vi "Channel Probe.vi"(2 "channelOp":enum16{"init", "write", "read", "probe"}(ring), 3 "PipeData in":refnum<class "StreamData.lvclass">) -> (1 "PipeData out":refnum<class "StreamData.lvclass">)   [LabVIEW 2017, in "Stream-t'WPI_EncoderType.ctl'.lvlib"]
doc: "Displays the status of the channel as the channel is modified by the various endpoints and gives the user ways to pause the application using the channel."
uses:
  <extravilib>/ChannelInstances/Stream-t'WPI_EncoderType.ctl'.lvlib
  <extravilib>/ChannelInstances/Stream-t'WPI_EncoderType.ctl'/StreamData.lvclass
  <vilib>/Rock Robotics/WPI/Encoder/WPI_EncoderType.ctl
  <extravilib>/ChannelInstances/Stream-t'WPI_EncoderType.ctl'/ChannelOp.ctl
  <vilib>/Utility/miscctls.llb/LVPositionTypeDef.ctl
panel:
  in  "Details":string="Details"
  in  "Operation Count":string="Operation Count:"
  out "Details":string
  in  "Last Operation":string="Last Operation:"
  in  "Read":string="Read"
  in  "Write":string="Write"
  in  "Single Step":bool
  in  "Element To Match":T1
  in  "Pause when latest element matches":bool
  in  "Pause when aborted":bool
  in  "Pause when last element written":bool
  in  "Fixed Size":string="<b>Current Element Count:</b>\n%d\n<b>Allocated Element Count:</b>\n%d (Fixed Size)\n"
  in  "Unbounded":string="<b>Current Element Count:</b>\n%d\n<b>Allocated Element Count:</b>\n%d (Unbounded)\n"
  out "Details":string
  in  "Play":bool
  out "Aborted?":bool
  out "Last element written?":bool
  in  "Pause":bool
  out "No Endpoiont Yet":string="\n\n\n\n\n\n\n\n\n\n\nNeither endpoint has executed yet."
  out "Latest":string="Latest\nEnqueue"
  out "Next":string="Next\nDequeue"
  out "Stream Data":cluster{"element":T1}[](array[cluster])
  # "Details"
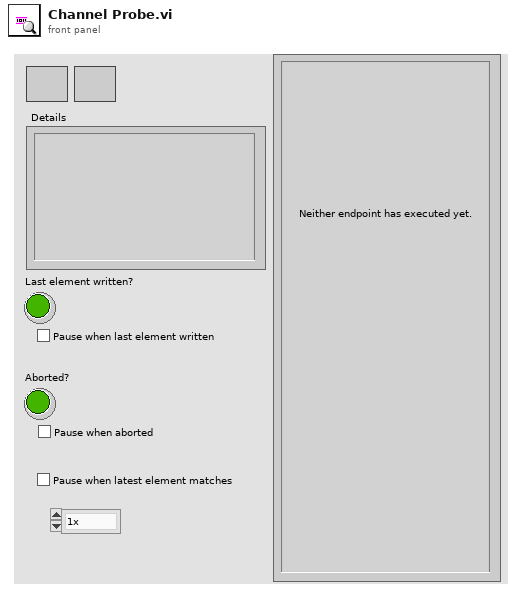
[diagram p1: front panel]
types:
  T1 = typedef "WPI_EncoderType.ctl" = enum16{"1x", "2x", "4x"}
  T2 = typedef "Stream-t'WPI_EncoderType.ctl'.lvlib/ChannelOp.ctl" = enum16{"init", "write", "read", "probe"}
  T3 = enum32{"Invalid", "Standard", "Closed", "Hidden", "Minimized", "Maximized"}
  T4 = typedef "LVPositionTypeDef.ctl" = cluster{"Left":i32, "Top":i32}
  T5 = typedef "LVPointTypeDef.ctl" = cluster{"Horizontal":i16, "Vertical":i16}
  T6 = typedef "LVBoundsTypeDef.ctl" = cluster{"Width":u32, "Height":u32}
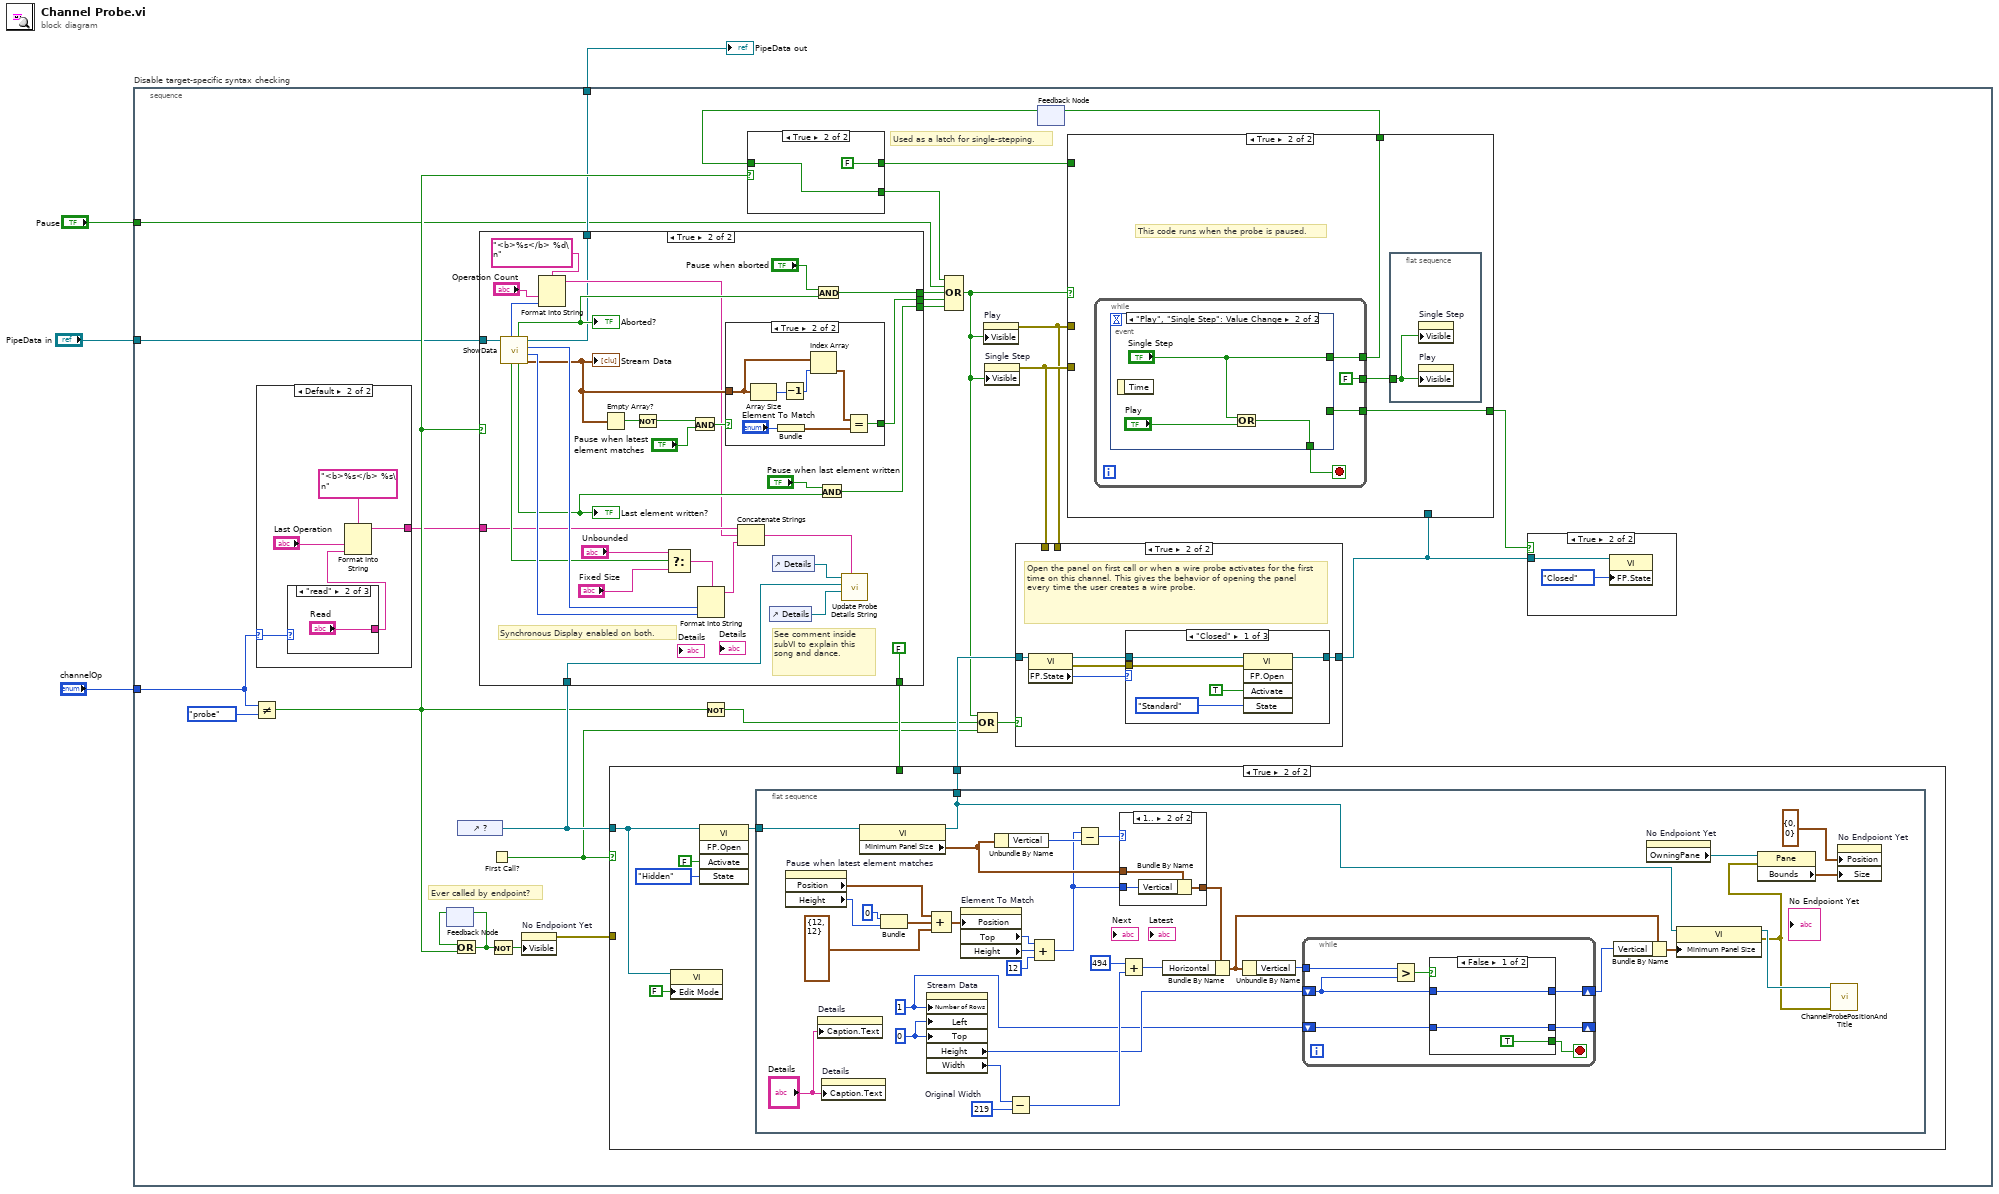
[diagram p0: block diagram]
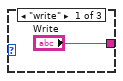
[diagram p3: hidden frame]
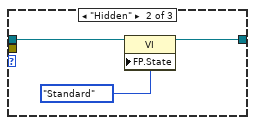
[diagram p7: hidden frame]
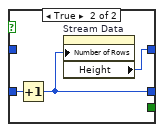
[diagram p12: hidden frame]
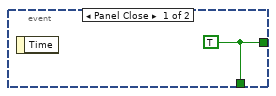
[diagram p15: hidden frame]
diagram:
  n1 = stacked-sequence "Disable target-specific syntax checking" {
    tunnel: "PipeData in" -> [w8]
    tunnel: [w7] -> w3
    tunnel: "Pause" -> [w6]
    tunnel: "channelOp" -> [w5]
    frame #0 {
      # "Used as a latch for single-stepping."
      # "Ever called by endpoint?"
      n2 = Not Equal?(x=w5, y=ChannelOp."probe" ("channelOp 2")) -> (x != y?=w15:bool)
      n3 = case shown="Default" w5 {
        selector: w5 -> [_ w38]
        tunnel: [_ w36] -> w11
        frame "init", "probe" {
        }
        frame Default {
          n4 = case shown="\"read\"" w38 {
            tunnel: ["Write" "Read" _] -> w35
            frame "write" {
            }
            frame "read" {
            }
            frame Default {
            }
          }
          n5 = Format Into String(format string="<b>%s</b> %s\n", "Last Operation", w35) -> (resulting string=w36:string)  [unwired: 2 in, 1 out]
        }
      }
      n6 = feedback #1() -> (w27:bool)  [unwired: 1 in]
      n7 = Or(x=w27, y=w15) -> (x .or. y?=w26:bool)
      n8 = feedback-in #1(w26) -> ()
      n9 = control-ref of="?"() -> (w28:refnum<vi>)
      n10 = case shown="True" w15 {
        tunnel: w8 -> [w59 w84]
        tunnel: [_ w79] -> w32
        tunnel: [_ w73] -> w31
        tunnel: [_ w72] -> w30
        tunnel: [_ FALSE ("always false")] -> w29
        tunnel: w28 -> [_ w70]
        tunnel: w11 -> [_ w69]
        tunnel: [w59 w60] -> w7
        frame False {
        }
        frame True {
          # "See comment inside subVI to explain this song and dance."
          # "Synchronous Display enabled on both."
          n11 = call <extravilib>:"ShowData.vi"("PipeData in"=w84) -> ("pipe data"=w77:cluster{"element":T1}[], "size"=w89:i32, "count"=w90:i32, "PipeData out"=w60:refnum<class "StreamData.lvclass">, "last element"=w83:bool, "abort"=w80:bool, "unbounded"=w88:bool, "OpCount"=w62:u32)  [unwired: 3 in]
          "Stream Data" <- w77
          "Last element written?" <- w83
          "Aborted?" <- w80
          n12 = Format Into String(format string="<b>%s</b> %d\n", "Operation Count", w62) -> (resulting string=w63:string)  [unwired: 2 in, 1 out]
          n13 = Empty Array?(array=w77) -> (empty?=w76:bool)
          n14 = Not(x=w76) -> (.not. x?=w75:bool)
          n15 = Select(t="Unbounded", s=w88, f="Fixed Size") -> (s? t:f=w85:string)
          n16 = And(x=w75, y="Pause when latest element matches") -> (x .and. y?=w74:bool)
          n17 = Format Into String(format string=w85, w90, w89) -> (resulting string=w64:string)  [unwired: 2 in, 1 out]
          n18 = case shown="True" w74 {
            tunnel: w77 -> [_ w94]
            tunnel: [_ w91] -> w73
            frame False {
            }
            frame True {
              n19 = Array Size(array=w94) -> (size(s)=w96:i32)
              n20 = Bundle("Element To Match"="Element To Match") -> (w92:cluster{"Element To Match":T1})  [unwired: 1 in]
              n21 = Decrement(x=w96) -> (x-1=w95:i32)
              n22 = Index Array(array=w94, index=w95) -> (element=w93:cluster{"element":T1})
              n23 = Equal?(x=w93, y=w92) -> (x = y?=w91:bool)
            }
          }
          n24 = Concatenate Strings(w69, w63, w64) -> (w66:string)
          n25 = control-ref of="Details"() -> (w71:refnum<vi>)
          n26 = control-ref of="Details"() -> (w68:refnum<vi>)
          n27 = And(x="Pause when aborted", y=w80) -> (x .and. y?=w79:bool)
          n28 = And(x="Pause when last element written", y=w83) -> (x .and. y?=w72:bool)
          n29 = call <resource>:"Update Probe Details String.vi"("String"=w66, "Details 1"=w71, "VI Reference"=w70, "Details 2"=w68) -> ()  [unwired: 8 in]
        }
      }
      n30 = First Call?() -> (First Call?: T/F=w13:bool)
      n31 = Not(x=w26) -> (.not. x?=w22:bool)
      n32 = property on="No Endpoiont Yet" class="Str"("Visible"=w22) -> (error out=w25:errorcluster)  [unwired: 2 in, 1 out]
      n33 = case shown="True" w13 {
        tunnel: [w98 w104] -> w23
        tunnel: w28 -> [w98 w100]
        tunnel: w29 -> [_ _]
        tunnel: w25 -> [_ _]
        frame False {
        }
        frame True {
          n34 = property class="VI"(reference=w100, "Edit Mode"=FALSE ("Edit Mode On Open")) -> ()  [unwired: 1 in, 2 out]
          n35 = invoke class="VI" method="FP.Open"(reference=w100, "Activate"=FALSE ("Activate?"), "State"=T3."Hidden") -> (reference out=w101:refnum<vi>)  [unwired: 2 in, 4 out]
          n36 = flat-sequence {
            tunnel: [w107] -> w104
            tunnel: w101 -> [w124]
            frame #0 {
              w113 = u32 1 ("Number of Rows")
              w121 = u32 219  # Original Width
              w123 = 0 ("Position:Top")
              n37 = property on="Pause when latest element matches" class="Bool (strict)"() -> ("Position"=w136:T4, "Height"=w138:u32)  [unwired: 2 in, 2 out]
              n38 = property on="Details" class="Str"("Caption.Text"="Details") -> ()  [unwired: 2 in, 2 out]
              n39 = property on="Details" class="Str"("Caption.Text"="Details") -> ()  [unwired: 2 in, 2 out]
              n40 = property class="VI"(reference=w124) -> (reference out=w107:refnum<vi>, "Minimum Panel Size"=w127:T5)  [unwired: 1 in, 1 out]
              n41 = Bundle("Bounds:Area Height"=u32 0, "Height"=w138) -> (w135:cluster{"Bounds:Area Height":u32, "Height":u32})  [unwired: 1 in]
              n42 = property on="Stream Data" class="Arr (strict)"("Number of Rows"=w113, "Left"=w123, "Top"=w123) -> ("Height"=w115:u32, "Width"=w122:u32)  [unwired: 2 in, 2 out]
              n43 = Compound Arithmetic op=ADD(w136, w135, T4 {"Left"=12, "Top"=12} ("Position")) -> (w133:cluster{u32, u32})
              n44 = property on="Element To Match" class="Enum (strict)"("Position"=w133) -> ("Top"=w132:i32, "Height"=w131:u32)  [unwired: 2 in, 2 out]
              n45 = Unbundle By Name(w127) -> ("Vertical"=w130:i16)
              n46 = Subtract(x=w122, y=w121) -> (x-y=w120:u32)
              n47 = Compound Arithmetic op=ADD(w132, w131, u32 12 ("value")) -> (w126:u32)
              n48 = Subtract(x=w126, y=w130) -> (x-y=w128:u32)
              n49 = case shown="1.." w128 {
                tunnel: w127 -> [w152 w155]
                tunnel: w126 -> [_ w154]
                tunnel: [w152 w153] -> w125
                frame Default {
                }
                frame 1.. {
                  n50 = Bundle By Name(cluster=w155, "Vertical"=w154) -> (w153:T5)
                }
              }
              n51 = Add(x=u32 494, y=w120) -> (x+y=w119:u32)
              n52 = Bundle By Name(cluster=w125, "Horizontal"=w119) -> (w117:T5)
              n53 = Unbundle By Name(w117) -> ("Vertical"=w118:i16)
              n54 = while {
                tunnel: w118 -> [w145]
                shift-right: [w142] -> _
                shift-left: w113 -> [w143]
                shift-right: [w140] -> w114
                shift-left: w115 -> [w139]
                stop <- w141 stop-if-true
                n55 = Greater?(x=w145, y=w139) -> (0:w144:bool)
                n56 = case shown="False" w144 {
                  tunnel: [TRUE _] -> w141
                  tunnel: w143 -> [w147 w151]
                  tunnel: [w147 w150] -> w142
                  tunnel: [w146 w149] -> w140
                  tunnel: w139 -> [w146 _]
                  frame False {
                  }
                  frame True {
                    n57 = Increment(x=w151) -> (x+1=w150:u32)
                    n58 = property on="Stream Data" class="Arr (strict)"("Number of Rows"=w150) -> ("Height"=w149:u32)  [unwired: 2 in, 2 out]
                  }
                }
              }
              n59 = Bundle By Name(cluster=w117, "Vertical"=w114) -> (w116:T5)
              n60 = property on="No Endpoiont Yet" class="Str"() -> ("OwningPane"=w111:refnum<vi>)  [unwired: 2 in, 2 out]
              n61 = property class="VI"(reference=w107, "Minimum Panel Size"=w116) -> (reference out=w106:refnum<vi>, error out=w105:errorcluster)  [unwired: 1 in]
              n62 = property class="Pane"(reference=w111, error in=w105) -> ("Bounds"=w110:T6)  [unwired: 2 out]
              n63 = call <resource>:"ChannelProbePositionAndTitle.vi"("error in (no error)"=w105, "VI in"=w106) -> ()  [unwired: 8 in, 2 out]
              n64 = property on="No Endpoiont Yet" class="Str"("Position"=T4 {"Left"=0, "Top"=0}, "Size"=w110) -> ()  [unwired: 2 in, 2 out]
            }
          }
        }
      }
      n65 = Not(x=w15) -> (.not. x?=w14:bool)
      n66 = feedback #2() -> (w20:bool)  [unwired: 1 in]
      n67 = case shown="True" w15 {
        tunnel: w20 -> [w41 w42]
        tunnel: [w41 FALSE] -> w19
        tunnel: [_ w42] -> w9
        frame False {
        }
        frame True {
        }
      }
      n68 = Compound Arithmetic op=OR(w9, w6, w32, w31, w30) -> (w10:bool)
      n69 = Compound Arithmetic op=OR(w10, w14, w13) -> (w12:bool)
      n70 = property on="Play" class="Bool"("Visible"=w10) -> (error out=w17:errorcluster)  [unwired: 2 in, 1 out]
      n71 = property on="Single Step" class="Bool"("Visible"=w10) -> (error out=w18:errorcluster)  [unwired: 2 in, 1 out]
      n72 = case shown="True" w12 {
        tunnel: [w44 w46] -> w24
        tunnel: w23 -> [w44 w45]
        tunnel: w18 -> [_ _]
        tunnel: w17 -> [_ _]
        frame False {
        }
        frame True {
          # "Open the panel on first call or when a wire probe activates for the first time on this channel. This gives the behavior of opening the panel every time the user creates a wire probe."
          n73 = property class="VI"(reference=w45) -> (reference out=w47:refnum<vi>, error out=w48:errorcluster, "FP.State"=w49:T3)  [unwired: 1 in]
          n74 = case shown="\"Closed\"" w49 {
            tunnel: w48 -> [w53 _ _]
            tunnel: w47 -> [w54 w57 w58]
            tunnel: [w50 w56 w58] -> w46
            frame "Closed" {
              n75 = invoke class="VI" method="FP.Open"(reference=w54, error in=w53, "Activate"=TRUE ("Activate?"), "State"=T3."Standard") -> (reference out=w50:refnum<vi>)  [unwired: 1 in, 4 out]
            }
            frame "Hidden" {
              n76 = property class="VI"(reference=w57, "FP.State"=T3."Standard" ("Front Panel Window:State")) -> (reference out=w56:refnum<vi>)  [unwired: 1 in, 1 out]
            }
            frame Default {
            }
          }
        }
      }
      n77 = case shown="True" w10 {
        tunnel: w24 -> [_ _]
        tunnel: [_ w159] -> w33
        tunnel: w17 -> [_ _]
        tunnel: w18 -> [_ _]
        tunnel: [w156 w157] -> w21
        tunnel: w19 -> [w156 _]
        frame False {
        }
        frame True {
          # "This code runs when the probe is paused."
          n78 = while {
            tunnel: [w164] -> w159
            tunnel: [FALSE ("Visible")] -> w158
            tunnel: [w161] -> w157
            stop <- w163 stop-if-true
            n79 = event shown="[1] \"Play\", \"Single Step\": Value Change" {
              selector: _ -> [_ _]
              dyn-events: _ -> [_ _]
              timeout: _ -> [_ _]
              tunnel: [w165 _] -> w164
              tunnel: [w165 w167] -> w163
              tunnel: [_ "Single Step"] -> w161
              event Panel Close {
                w165 = TRUE
                n80 = event-data() -> ()  [unwired: 1 in, 1 out]
              }
              event "Play", "Single Step": Value Change {
                n81 = event-data() -> ()  [unwired: 1 in, 1 out]
                n82 = Or(x="Single Step", y="Play") -> (x .or. y?=w167:bool)
              }
            }
          }
          n83 = flat-sequence {
            tunnel: w158 -> [w160]
            frame #0 {
              n84 = property on="Single Step" class="Bool"("Visible"=w160) -> ()  [unwired: 2 in, 2 out]
              n85 = property on="Play" class="Bool"("Visible"=w160) -> ()  [unwired: 2 in, 2 out]
            }
          }
        }
      }
      n86 = feedback-in #2(w21) -> ()
      n87 = case shown="True" w33 {
        tunnel: w24 -> [_ w169]
        frame False {
        }
        frame True {
          n88 = property class="VI"(reference=w169, "FP.State"=T3."Closed" ("Front Panel Window:State")) -> ()  [unwired: 1 in, 2 out]
        }
      }
    }
  }
  "PipeData out" <- w3
